vi "FTW-JSON-Object-SetElement-Integer.vi"(0 "JSON Object":refnum<class "FTW-JSON.lvclass">, 5 "Key":string, 7 "Value":i32, 11 "error in":errorcluster) -> (4 "JSON Object out":refnum<class "FTW-JSON.lvclass">, 15 "error out":errorcluster)   [LabVIEW 2013, in "FTW-JSON.lvclass"]
uses:
  FTW-JSON.lvclass
  FTW-JSON.lvclass/FTW-JSON.ctl
panel:
  # "Inputs"
  # "Outputs"
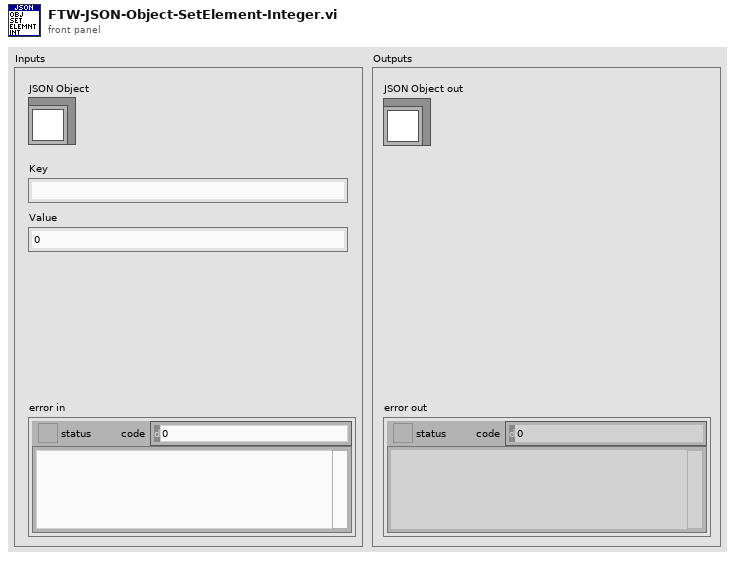
[diagram p1: front panel]
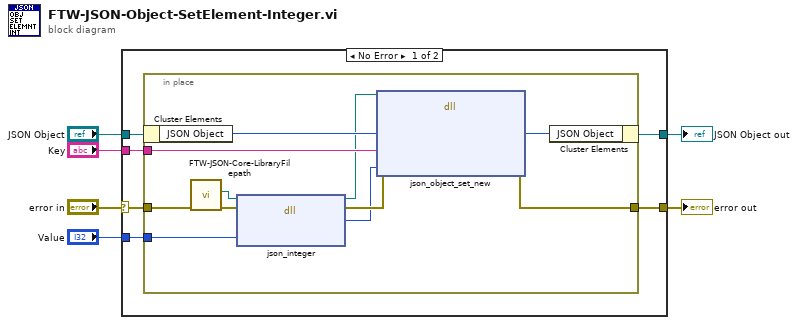
[diagram p0: block diagram]
diagram:
  n1 = case shown="No Error" "error in" {
    selector: "error in" -> [w12 w25]
    tunnel: [w11 w25] -> w6
    tunnel: [w9 w24] -> w4
    tunnel: "JSON Object" -> [w10 w24]
    tunnel: "Key" -> [w8 _]
    tunnel: "Value" -> [w7 _]
    frame No Error {
      n2 = in-place {
        in-place-border: w12 -> [w23]
        in-place-border: [w22] -> w11
        in-place-border: w8 -> [w19]
        in-place-border: w7 -> [w14]
        n3 = in-place-cluster #1(w10) -> ("JSON Object"=w21:i64)
        n4 = call "FTW-JSON-Core-LibraryFilepath.vi"("error in"=w23) -> ("error out"=w16:errorcluster, "JSON Library Filepath"=w18:path)  [unwired: 9 in]
        n5 = dll-call lib="?" fn="json_integer"(path in=w18, error in=w16, "I32 Value"=w14) -> (path out=w17:path, error out=w15:errorcluster, "New Double Value"=w13:i64)  [unwired: 2 in]
        n6 = dll-call lib="?" fn="json_object_set_new"(path in=w17, error in=w15, "JSON Object Pointer"=w21, "Key"=w19, "New JSON Object"=w13) -> (error out=w22:errorcluster, "JSON Object Pointer"=w20:i64)  [unwired: 4 in, 1 out]
        n7 = in-place-cluster #1("JSON Object"=w20) -> (w9:refnum<class "FTW-JSON.lvclass">)
      }
    }
    frame Error {
    }
  }
  "error out" <- w6
  "JSON Object out" <- w4
